vi "setSubtype.vi"(8 "error in (no error)":errorcluster, 10 "Type":T1 items=["Generic"=0, "Function"=1, "Binary (Old)"=2, "UUID"=3, "MD5"=5, "User Defined"=128], 11 "tBSONBinary in":refnum<class "tBSONBinary.lvclass">) -> (0 "error out":errorcluster, 3 "tBSONBinary out":refnum<class "tBSONBinary.lvclass">)   [LabVIEW 2013, in "BSON.lvlib" / "tBSONBinary.lvclass"]
uses:
  tBSONBinary.lvclass
  Subtype.ctl
  tBSONBinary.lvclass/tBSONBinary.ctl
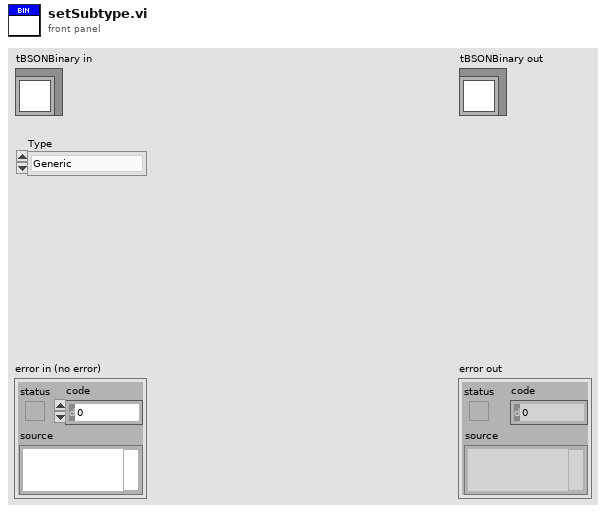
[diagram p1: front panel]
types:
  T1 = typedef "BSON.lvlib/tBSONBinary.lvclass/Subtype.ctl" = u8
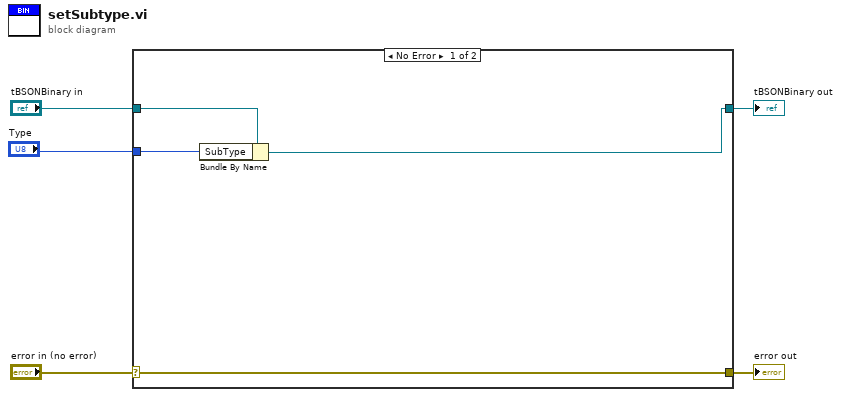
[diagram p0: block diagram]
diagram:
  n1 = case shown="No Error" "error in (no error)" {
    selector: "error in (no error)" -> [w9 w11]
    tunnel: [w9 w11] -> w4
    tunnel: [w6 w10] -> w2
    tunnel: "tBSONBinary in" -> [w8 w10]
    tunnel: "Type" -> [w7 _]
    frame No Error {
      n2 = Bundle By Name(cluster=w8, "SubType"=w7) -> (w6:refnum<class "tBSONBinary.lvclass">)
    }
    frame Error {
    }
  }
  "error out" <- w4
  "tBSONBinary out" <- w2
